vi "Generate Report as INI Section.vi"(7 "Parameters":variant, 8 "error in (no error)":errorcluster, 9 "Results":variant, 10 "Refnum in":T1, 11 "Analyze Fluence in":refnum<class "Analyze Fluence.lvclass">) -> (0 "error out":errorcluster, 2 "Refnum out":T1, 3 "Analyze Fluence out":refnum<class "Analyze Fluence.lvclass">)   [LabVIEW 2009, in "Analyze Fluence.lvclass"]
uses:
  Analyze Fluence.lvclass
  <vilib>/Utility/config.llb/Config Data RefNum.ctl
  <vilib>/Utility/config.llb/Write Key (Double).vi
  <vilib>/Utility/config.llb/NI_LVConfig.lvlib
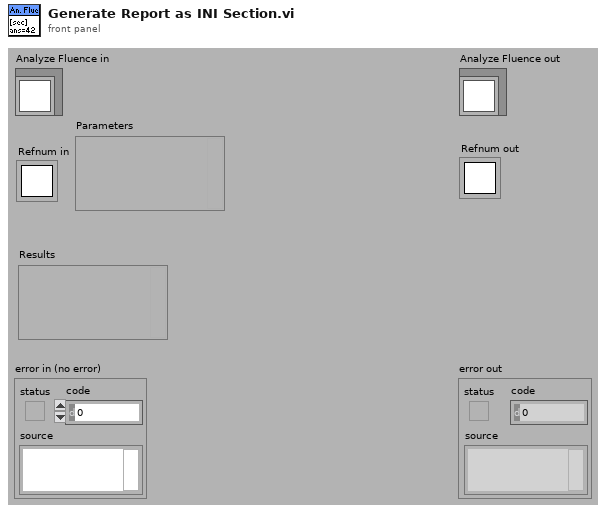
[diagram p1: front panel]
types:
  T1 = typedef "NI_LVConfig.lvlib/Config Data RefNum.ctl" = refnum<k1>
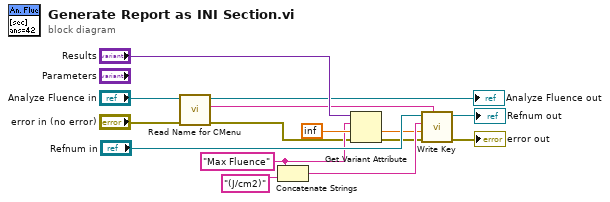
[diagram p0: block diagram]
diagram:
  w7 = "Max Fluence" ("name")
  n1 = call-dynamic "Read Name for CMenu.vi"("error in (no error)"="error in (no error)", "Analyze BaseClass in"="Analyze Fluence in") -> ("error out"=w2:errorcluster, "Name for Context menu"=w9:string, "Analyze BaseClass out"=→"Analyze Fluence out":refnum<class "Analyze Fluence.lvclass">)  [unwired: 7 in]
  n2 = Concatenate Strings(w7, "(J/cm2)" ("string")) -> (w6:string)
  n3 = Get Variant Attribute(Variant="Results", name=w7, default value (empty Variant)=inf, error in=w2) -> (value=w3:dbl, error out=w1:errorcluster)  [unwired: 2 out]
  n4 = call-poly <vilib>:"Write Key.vi"("section"=w9, "error in (no error)"=w1, "value"=w3, "key"=w6, "refnum"="Refnum in") -> ("error out"=→"error out":errorcluster, "refnum out"=→"Refnum out":T1)  [unwired: 4 in, 1 out]
